vi "Get Children Recursively.vi"(2 "error in":errorcluster, 3 "Parent":string, 4 "Tree":refnum<vi>) -> (0 "error out":errorcluster, 1 "Recursive Children":string[](array[string]))   [LabVIEW 2011, in "GraphicalTestRunner.lvlib"]
uses:
  GraphicalTestRunner.lvlib
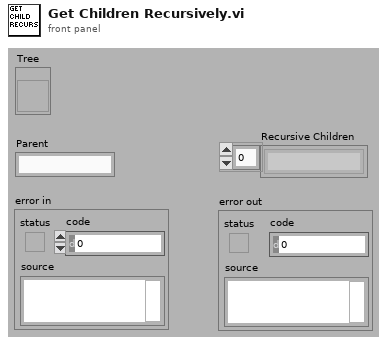
[diagram p1: front panel]
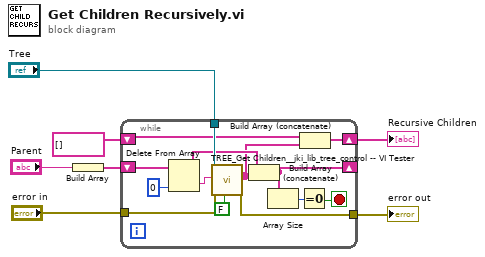
[diagram p0: block diagram]
diagram:
  n1 = Build Array("Parent") -> (w6:string[])
  n2 = while {
    shift-right: [w15] -> _
    shift-left: w6 -> [w12]
    tunnel: "Tree" -> [w19]
    tunnel: "error in" -> [w18]
    tunnel: [w17] -> w3
    shift-right: [w8] -> w5
    shift-left: string[] [] ("appended array") -> [w10]
    stop <- w13 stop-if-true
    n3 = Delete From Array(array=w12, index=0) -> (deleted portion=w20:string, array with subset deleted=w16:string[])  [unwired: 1 in]
    n4 = call "TREE_Get Children__jki_lib_tree_control -- VI Tester.vi"("Tree Reference In"=w19, "Parent Tag"=w20, "error in (no error)"=w18, "Use Current"=FALSE) -> ("Children Tags"=w9:string[], "error out"=w17:errorcluster)  [unwired: 13 in, 1 out]
    n5 = Build Array (concatenate)(w16, w9) -> (w15:string[])
    n6 = Array Size(array=w15) -> (size(s)=w14:i32)
    n7 = Equal To 0?(x=w14) -> (x = 0?=w13:bool)
    n8 = Build Array (concatenate)(w10, w9) -> (w8:string[])
  }
  "Recursive Children" <- w5
  "error out" <- w3
